vi "Z_switch_heating.vi"(10 "Z":T2={"Z_HSw"=1, "Z_HSetState"=enum."on", "Z_ASetState"=enum."on", "Z_DSetState"=enum."on"}, 11 "Z_LSw":u32=2) -> (2 "Z_SetState":T1=enum."on", 3 "Z_Source":T3=enum."local disabled")   [LabVIEW 2019, in "Heating.lvlib"]
uses:
  Heating.lvlib
  ctl/Z_State.ctl
  ctl/Y_source.ctl
panel:
  # "Входы\nZ_LSw – переключатель р/а. 1 приоритет\n     0 – откл\n     1 – ручной (местный)\n     2 – автомат\nZ_HSw – источник управления из меню. 2 приоритет\n     0 – ручной контроллера\n     1 – автомат контроллера\n     2 – дистационный\nZ_HSetState – заданное состояние в меню или на панели\nZ_ASetState – заданное состояние от вышестоящего алгоритма\nZ_DSetState – заданное состояние дистанционно\n     1 – alarm (авария)\n     2 – disabled (выведен из работы)\n     4 – stop (стоп - готов к работе)\n     5 – reserv (резерв)\n     9 – check (проверка работоспособности)\n     10 – on min (включен на минимуме)\n     12 – on (включен)\n     14 – on max (включен на максимуме)\n     15... -> 3 – стоп"
  # "Выходы\nZ_Source – источник управления:\n     0 – initialize (Инициализация)\n     1 – local disabled (Выведен из работы по месту)\n     2 – local hand (Ручной местный)\n     3 – hand (Ручной контроллера)\n     4 – auto (Автомат контроллера)\n     5 – dist (Дистанционный)\nZ_SetState(Z2) - состояние автомата механизма:\n     1 – alarm (авария)\n     2 – disabled (выведен из работы)\n     4 – stop (стоп - готов к работе)\n     5 – reserv (резерв)\n     9 – check (проверка работоспособности)\n     10 – on min (включен на минимуме)\n     12 – on (включен)\n     14 – on max (включен на максимуме)"
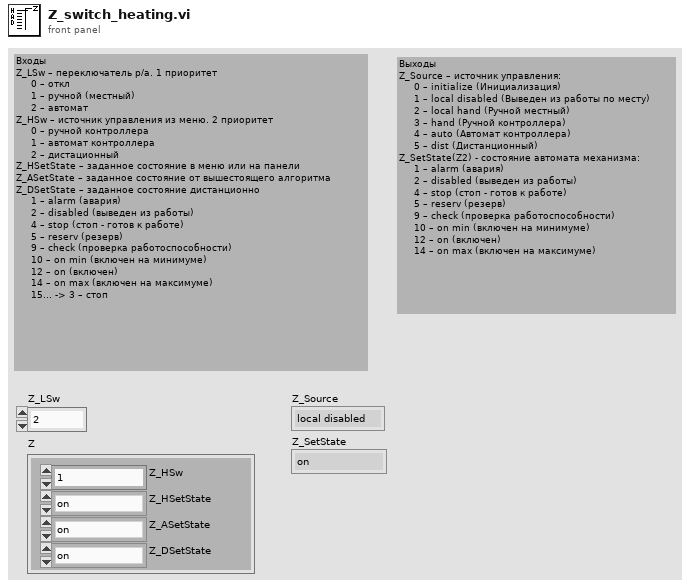
[diagram p1: front panel]
types:
  T1 = typedef "Heating.lvlib/Z_State.ctl" = enum8{"initialization", "alarm", "disabled", "not ready", "stop ready", "reserv", "switched off", "reserv2", "switched on", "check", "on min", "decrease out", "on", "increase out", "on max"}
  T2 = cluster{"Z_HSw":u32, "Z_HSetState":T1, "Z_ASetState":T1, "Z_DSetState":T1}
  T3 = typedef "Heating.lvlib/Y_source.ctl" = enum8{"initialize", "local disabled", "local hand", "hand", "auto", "dist"}
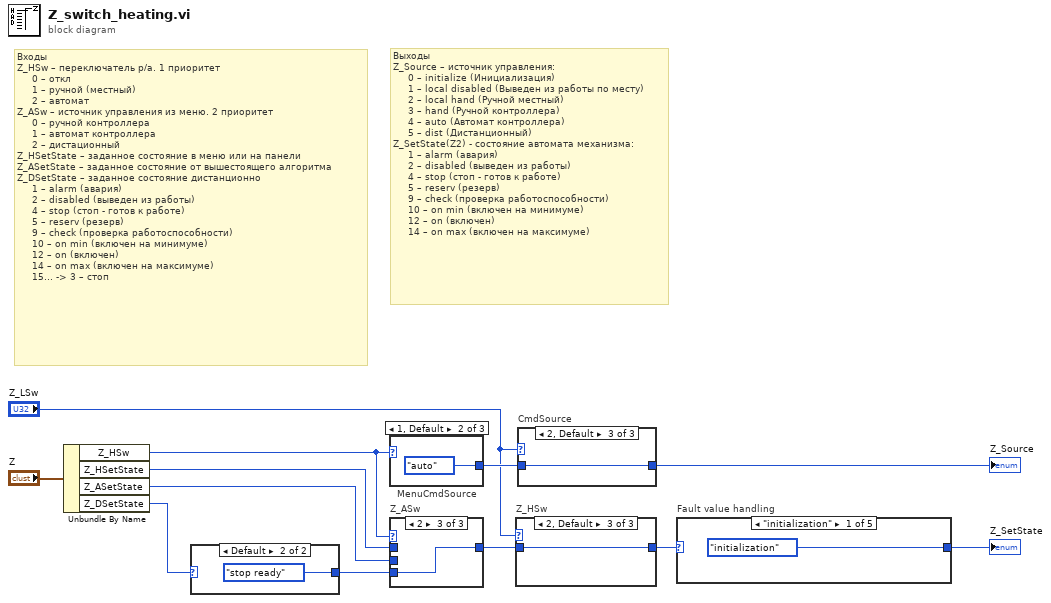
[diagram p0: block diagram]
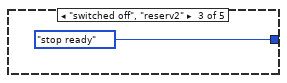
[diagram p3: hidden frame]
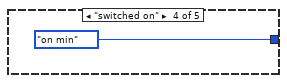
[diagram p4: hidden frame]
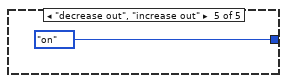
[diagram p5: hidden frame]
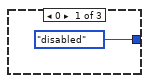
[diagram p9: hidden frame]
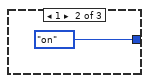
[diagram p10: hidden frame]
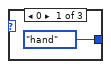
[diagram p11: hidden frame]
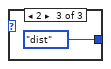
[diagram p12: hidden frame]
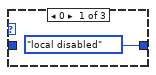
[diagram p13: hidden frame]
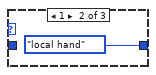
[diagram p14: hidden frame]
diagram:
  # "Входы\nZ_HSw – переключатель р/а. 1 приоритет\n     0 – откл\n     1 – ручной (местный)\n     2 – автомат\nZ_ASw – источник управления из меню. 2 приоритет\n     0 – ручной контроллера\n     1 – автомат контроллера\n     2 – дистационный\nZ_HSetState – заданное состояние в меню или на панели\nZ_ASetState – заданное состояние от вышестоящего алгоритма\nZ_DSetState – заданное состояние дистанционно\n     1 – alarm (авария)\n     2 – disabled (выведен из работы)\n     4 – stop (стоп - готов к работе)\n     5 – reserv (резерв)\n     9 – check (проверка работоспособности)\n     10 – on min (включен на минимуме)\n     12 – on (включен)\n     14 – on max (включен на максимуме)\n     15... -> 3 – стоп"
  # "Выходы\nZ_Source – источник управления:\n     0 – initialize (Инициализация)\n     1 – local disabled (Выведен из работы по месту)\n     2 – local hand (Ручной местный)\n     3 – hand (Ручной контроллера)\n     4 – auto (Автомат контроллера)\n     5 – dist (Дистанционный)\nZ_SetState(Z2) - состояние автомата механизма:\n     1 – alarm (авария)\n     2 – disabled (выведен из работы)\n     4 – stop (стоп - готов к работе)\n     5 – reserv (резерв)\n     9 – check (проверка работоспособности)\n     10 – on min (включен на минимуме)\n     12 – on (включен)\n     14 – on max (включен на максимуме)"
  n1 = Unbundle By Name("Z") -> ("Z_HSw"=w4:u32, "Z_HSetState"=w3:T1, "Z_ASetState"=w2:T1, "Z_DSetState"=w1:T1)
  n2 = case shown="Default" w1 {
    selector: w1 -> [w13 _]
    tunnel: [w13 Z_State."stop ready" ("X5(DistSetSate) 2")] -> w8
    frame "alarm".."on max" {
    }
    frame Default {
    }
  }
  n3 = case "MenuCmdSource" shown="1, Default" w4 {
    tunnel: [Y_source."hand" ("Z1(CmdSource) 3") Y_source."auto" ("Z1(CmdSource) 3") Y_source."dist" ("Z1(CmdSource) 3")] -> w12
    frame 0 {
    }
    frame 1, Default {
    }
    frame 2 {
    }
  }
  n4 = case "Z_ASw" shown="2" w4 {
    tunnel: [w18 w19 w20] -> w10
    tunnel: w3 -> [w18 _ _]
    tunnel: w8 -> [_ _ w20]
    tunnel: w2 -> [_ w19 _]
    frame 0 {
    }
    frame 1, Default {
    }
    frame 2 {
    }
  }
  n5 = case "Z_HSw" shown="2, Default" "Z_LSw" {
    tunnel: [Z_State."disabled" ("X5(DistSetSate) 2") Z_State."on" ("X5(DistSetSate) 2") w23] -> w9
    tunnel: w10 -> [_ _ w23]
    frame 0 {
    }
    frame 1 {
    }
    frame 2, Default {
    }
  }
  n6 = case "CmdSource" shown="2, Default" "Z_LSw" {
    tunnel: [Y_source."local disabled" ("Z1(CmdSource) 3") Y_source."local hand" ("Z1(CmdSource) 3") w26] -> w6
    tunnel: w12 -> [_ _ w26]
    frame 0 {
    }
    frame 1 {
    }
    frame 2, Default {
    }
  }
  "Z_Source" <- w6
  n7 = case "Fault value handling" shown="\"initialization\"" w9 {
    selector: w9 -> [_ w28 _ _ _]
    tunnel: [Z_State."initialization" ("X5(DistSetSate) 2") w28 Z_State."stop ready" ("X5(DistSetSate) 2") Z_State."on min" ("X5(DistSetSate) 2") Z_State."on" ("X5(DistSetSate) 2")] -> w7
    frame "initialization" {
    }
    frame "alarm".."reserv", "check", "on", "on max", Default {
    }
    frame "switched off", "reserv2" {
    }
    frame "switched on" {
    }
    frame "decrease out", "increase out" {
    }
  }
  "Z_SetState" <- w7
